vi "FIR_5decimate_5cycles_32bit_for_5761.vi"(7 "reset":bool, 8 "valid in":bool, 10 "Q in":fxp<+/-,32,14>, 11 "I in":fxp<+/-,32,14>) -> (0 "valid out":bool, 2 "Q out":fxp<+/-,32,14>, 3 "I out":fxp<+/-,32,14>, 4 "ready for input":bool)   [LabVIEW 2025]
uses:
  <vilib>/rvi/IPIntegrationNode/IPINode_Typedef/niFpgaIPINodeSupportedFamilies.ctl
  <vilib>/rvi/FXPMathLib/FxpConvert/subVIs/nifxpmath_Convert_SimConfig.ctl
  <vilib>/fxp/LVFixedPointQuantizationPolicyTypeDef.ctl
  <vilib>/fxp/LVFixedPointOverflowPolicyTypeDef.ctl
  <vilib>/rvi/IPIntegrationNode/IPINode_Utilities/niFpgaIPINodeSimCore.vi
  <vilib>/rvi/FXPMathLib/FxpConvert/simVIs/DllFxpConvertTemp_sub.vi
  <vilib>/rvi/XilinxIP/XIPIN_XNode/niFpgaXIPIN.xnode
  FIR_5decimate_5cycles_32bit_for_5761/xsim.dir/FIR_5decimate_5cycles_32bit_for_5761_068759B7C2FC41C097D7805413A434EE/xsimk_068759B7C2FC41C097D7805413A434EE.dll
  <vilib>/rvi/IPIntegrationNode/IPINode_Xnode/niFpgaIPINode.xnode
  <vilib>/rvi/FXPMathLib/FxpInterpret/XNode/nifxpmath_Interpret.xnode
  <vilib>/rvi/FXPMathLib/FxpConvert/XNode/nifxpmath_Convert.xnode
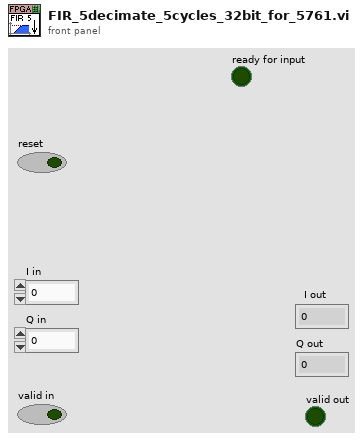
[diagram p1: front panel]
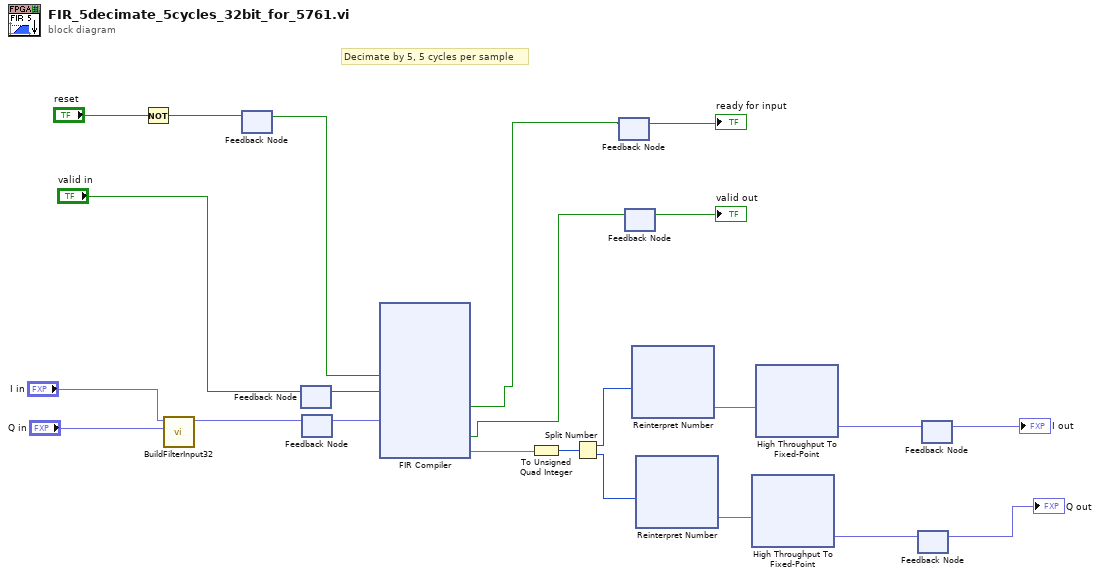
[diagram p0: block diagram]
diagram:
  # "Decimate by 5, 5 cycles per sample"
  n1 = Not(x="reset") -> (.not. x?=w16:bool)
  n2 = call "BuildFilterInput32.vi"("Q in"="Q in", "I in"="I in") -> ("Filter input"=w7:fxp<+,64,64>)  [unwired: 9 in]
  n3 = feedback #1() -> (w6:bool)  [unwired: 1 in]
  n4 = feedback-in #1(w16) -> ()
  n5 = feedback #2() -> (w5:bool)  [unwired: 1 in]
  n6 = feedback-in #2("valid in") -> ()
  n7 = feedback-in #3(w7) -> ()
  n8 = feedback #3() -> (w4:fxp<+,64,64>)  [unwired: 1 in]
  n9 = xnode ("FIR Compiler")("aresetn"=w6, "s_axis_data_tvalid"=w5, "s_axis_data_tdata"=w4) -> ("s_axis_data_tready"=w3:bool, "m_axis_data_tvalid"=w1:bool, "m_axis_data_tdata"=w2:fxp<+,64,64>)  [unwired: 1 in]
  n10 = To Unsigned Quad Integer(1:w2) -> (0:w21:u64)
  n11 = Split Number(x=w21) -> (hi(x)=w22:u32, lo(x)=w18:u32)
  n12 = feedback #4() -> (→"ready for input":bool)  [unwired: 1 in]
  n13 = feedback-in #4(w3) -> ()
  n14 = feedback #5() -> (→"valid out":bool)  [unwired: 1 in]
  n15 = feedback-in #5(w1) -> ()
  n16 = xnode "Reinterpret Number"("x"=w22) -> ("y"=w19:fxp<+/-,32,15>)
  n17 = xnode "Reinterpret Number"("x"=w18) -> ("y"=w20:fxp<+/-,32,15>)
  n18 = xnode "High Throughput To Fixed-Point"("x"=w20) -> ("y"=w13:fxp<+/-,32,14>)
  n19 = xnode "High Throughput To Fixed-Point"("x"=w19) -> ("y"=w15:fxp<+/-,32,14>)
  n20 = feedback #6() -> (→"Q out":fxp<+/-,32,14>)  [unwired: 1 in]
  n21 = feedback-in #6(w13) -> ()
  n22 = feedback #7() -> (→"I out":fxp<+/-,32,14>)  [unwired: 1 in]
  n23 = feedback-in #7(w15) -> ()
